vi "check bakground and image are same size.vi"(10 "background array":u16[][](array[numeric]), 11 "image array":u16[][](array[numeric])) -> (3 "background array out":u16[][](array[numeric]))   [LabVIEW 2020, in "Point Grey Camera.lvclass"]
uses:
  Point Grey Camera.lvclass
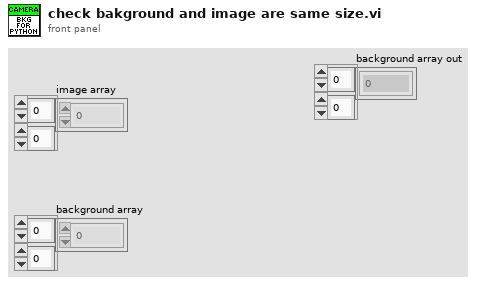
[diagram p1: front panel]
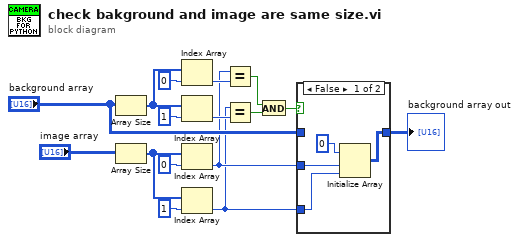
[diagram p0: block diagram]
diagram:
  n1 = Array Size(array="background array") -> (size(s)=w14:i32[])
  n2 = Array Size(array="image array") -> (size(s)=w13:i32[])
  n3 = Index Array(array=w14, index=0) -> (element=w9:i32)
  n4 = Index Array(array=w14, index=1) -> (element=w12:i32)
  n5 = Index Array(array=w13, index=0) -> (element=w2:i32)
  n6 = Index Array(array=w13, index=1) -> (element=w1:i32)
  n7 = Equal?(x=w2, y=w9) -> (x = y?=w15:bool)
  n8 = Equal?(x=w1, y=w12) -> (x = y?=w16:bool)
  n9 = And(x=w15, y=w16) -> (x .and. y?=w5:bool)
  n10 = case shown="False" w5 {
    tunnel: "background array" -> [_ w21]
    tunnel: [w17 w21] -> w3
    tunnel: w2 -> [w19 _]
    tunnel: w1 -> [w18 _]
    frame False {
      n11 = Initialize Array(u16 0, w19, w18) -> (w17:u16[][])
    }
    frame True {
    }
  }
  "background array out" <- w3
